vi "Boiler Controller.vi"(8 "error in (no error)":errorcluster, 11 "Message Queues":T1) -> (0 "error out":errorcluster)   [LabVIEW 2015]
uses:
  support/Message Queue/All Message Queues.ctl
  support/Message Queue/Message Cluster.ctl
  support/Message Queue/Message Queue.lvlib
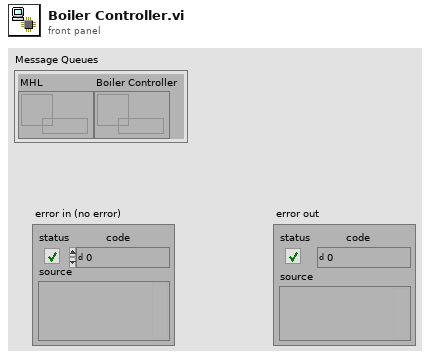
[diagram p1: front panel]
types:
  T1 = typedef "Message Queue.lvlib/All Message Queues.ctl" = cluster{"MHL":refnum<queue>, "Boiler Controller":refnum<queue>}
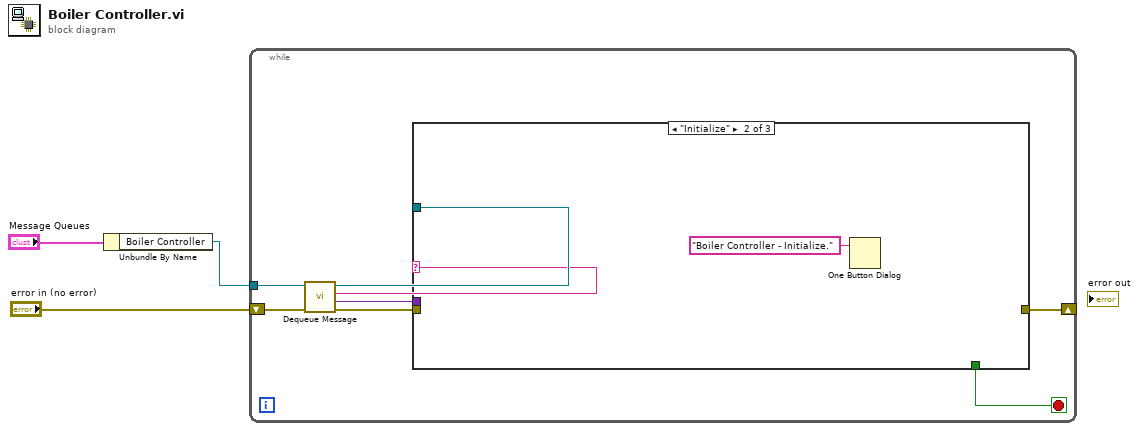
[diagram p0: block diagram]
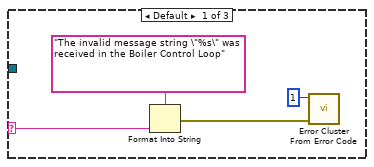
[diagram p2: hidden frame]
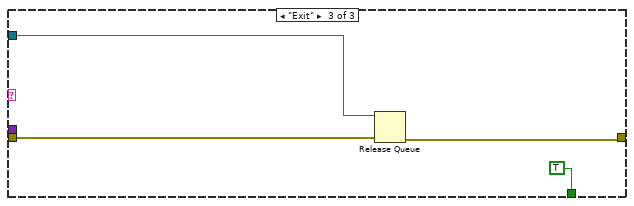
[diagram p3: hidden frame]
diagram:
  n1 = Unbundle By Name("Message Queues") -> ("Boiler Controller"=w1:refnum<queue>)
  n2 = while {
    shift-right: [w5] -> _
    shift-left: "error in (no error)" -> [w11]
    tunnel: w1 -> [w10]
    stop <- w4 stop-if-true
    n3 = call "Dequeue Message.vi"("error in (no error)"=w11, "Message Queue"=w10) -> ("error out"=w7:errorcluster, "Message Data"=w6:variant, "Message"=w8:string, "dup Message Queue"=w9:refnum<queue>)  [unwired: 6 in]
    n4 = case shown="\"Initialize\"" w8 {
      selector: w8 -> [w15 _ _]
      tunnel: w9 -> [_ _ w17]
      tunnel: w7 -> [_ _ w19]
      tunnel: w6 -> [_ _ _]
      tunnel: [_ _ w18] -> w5
      tunnel: [_ _ TRUE] -> w4
      frame Default {
        n5 = Format Into String(format string="The invalid message string \"%s\" was received in the Boiler Control Loop", w15) -> (error out=w13:errorcluster)  [unwired: 2 in, 1 out]
        n6 = call <vilib>:"Error Cluster From Error Code.vi"("error in (no error)"=w13, "error code (0)"=1) -> ()  [unwired: 7 in, 1 out]
      }
      frame "Initialize" {
        n7 = One Button Dialog(message="Boiler Controller - Initialize.") -> ()  [unwired: 1 in, 1 out]
      }
      frame "Exit" {
        n8 = Release Queue(queue=w17, error in (no error)=w19) -> (error out=w18:errorcluster)  [unwired: 1 in, 2 out]
      }
    }
  }
